vi "LS370_Check_Queue.vi"(7 "error in (no error)":errorcluster, 10 "queue":refnum<queue>) -> (0 "error out":errorcluster, 1 "Control":T1, 3 "New Entries?":bool)   [LabVIEW 2019]
uses:
  LS370/LS370-Control.ctl
panel:
  out "Numeric":i32
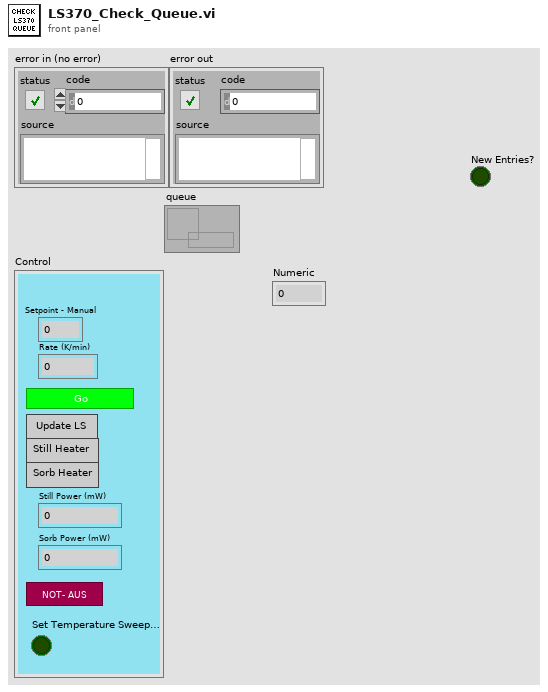
[diagram p1: front panel]
types:
  T1 = typedef "LS370-Control.ctl" = cluster{"Disable Heater":bool, "Activate Tsweep":bool, "Update Lakeshores":bool, "Setpoint - Manual":dbl, "Rate (K/min)":dbl, "Sorb Power (mW)":dbl, "Still Power (mW)":dbl, "Sorb Heater":bool, "Still Heater":bool, "Set Temperature Sweep Main":bool}
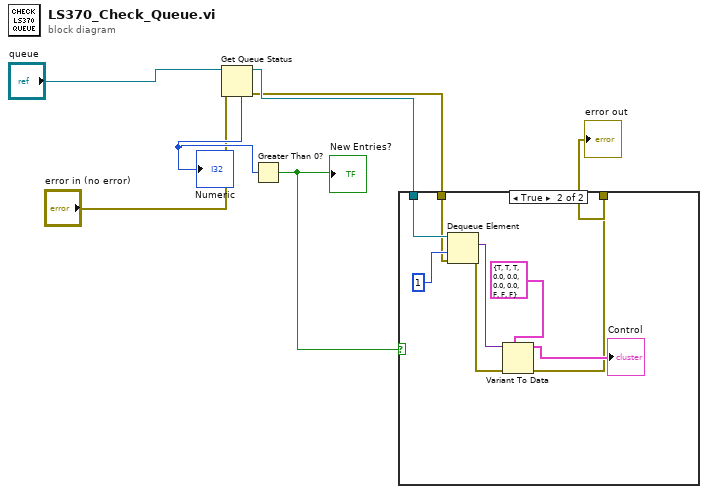
[diagram p0: block diagram]
diagram:
  n1 = Get Queue Status(queue="queue", error in (no error)="error in (no error)") -> (queue out=w6:refnum<queue>, error out=w4:errorcluster, # elements in queue=w7:i32)  [unwired: 1 in, 5 out]
  "Numeric" <- w7
  n2 = Greater Than 0?(x=w7) -> (x > 0?=w5:bool)
  "New Entries?" <- w5
  n3 = case shown="True" w5 {
    tunnel: w6 -> [_ w13]
    tunnel: w4 -> [w8 w11]
    tunnel: [w8 w9] -> w2
    frame False {
    }
    frame True {
      n4 = Dequeue Element(queue=w13, timeout in ms (-1)=1, error in (no error)=w11) -> (element=w15:variant, error out=w10:errorcluster)  [unwired: 2 out]
      n5 = Variant To Data(error in=w10, type=T1 {"Disable Heater"=TRUE, "Activate Tsweep"=TRUE, "Update Lakeshores"=TRUE, "Setpoint - Manual"=0.0, "Rate (K/min)"=0.0, "Sorb Power (mW)"=0.0, "Still Power (mW)"=0.0, "Sorb Heater"=FALSE, "Still Heater"=FALSE, "Set Temperature Sweep Main"=FALSE} ("JT-Cluster"), Variant=w15) -> (data=→"Control":T1, error out=w9:errorcluster)
    }
  }
  "error out" <- w2
